vi "Add Snake Class.vi"(8 "error in (no error)":errorcluster, 10 "Snake":refnum<class "Snake.lvclass">, 11 "Board_Game in":refnum<class "Board_Game.lvclass">) -> (0 "error out":errorcluster, 3 "Board_Game out":refnum<class "Board_Game.lvclass">)   [LabVIEW 2021, in "Board_Game.lvclass"]
uses:
  Board_Game.lvclass
  SnakeGame/Snake.lvclass
  Direction.ctl
  Board_Game.lvclass/Board_Game.ctl
  SnakeGame/Position.ctl
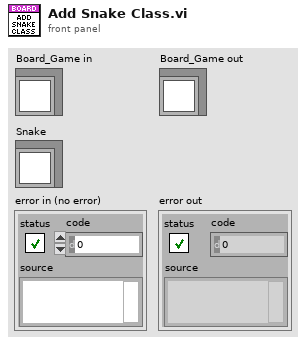
[diagram p1: front panel]
types:
  T1 = typedef "Direction.ctl" = enum16{"Up", "Down", "Left", "Right"}
  T2 = typedef "Position.ctl" = cluster{"X":u32, "Y":u32}
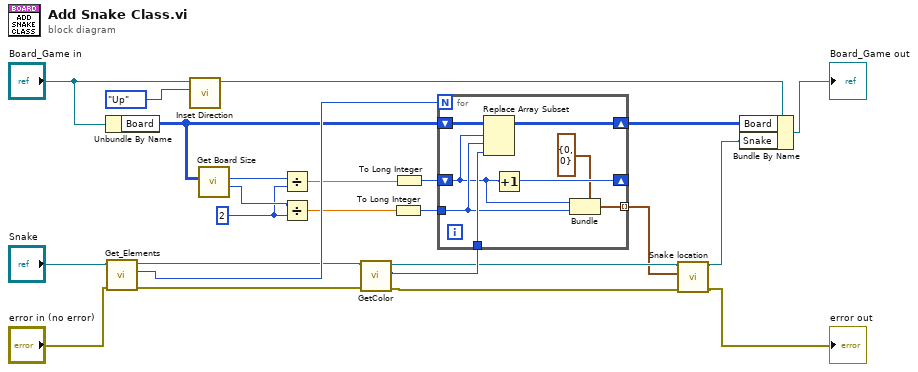
[diagram p0: block diagram]
diagram:
  w8 = 2 ("y")
  n1 = Unbundle By Name("Board_Game in") -> ("Board"=w13:u32[][])
  n2 = call-dynamic "Get_Elements.vi"("error in (no error)"="error in (no error)", "Snake in"="Snake") -> ("error out"=w5:errorcluster, "Start Elements"=w17:u32, "Snake out"=w16:refnum<class "Snake.lvclass">)  [unwired: 7 in]
  n3 = call-dynamic "Inset Direction.vi"("Keyboard"=Direction."Up", "Board_Game in"="Board_Game in") -> ("Board_Game out"=w22:refnum<class "Board_Game.lvclass">)  [unwired: 8 in, 1 out]
  n4 = call "Get Board Size.vi"("Board"=w13) -> ("Y"=w9:i32, "X"=w12:i32)  [unwired: 9 in]
  n5 = Divide(x=w12, y=w8) -> (x/y=w11:dbl)
  n6 = Divide(x=w9, y=w8) -> (x/y=w10:dbl)
  n7 = call-dynamic "GetColor.vi"("error in (no error)"=w5, "SnakeGame in"=w16) -> ("error out"=w3:errorcluster, "Color"=w14:u32, "SnakeGame out"=w7:refnum<class "Snake.lvclass">)  [unwired: 7 in]
  n8 = To Long Integer(number=w10) -> (32bit integer=w18:i32)
  n9 = To Long Integer(number=w11) -> (32bit integer=w19:i32)
  n10 = for {
    N: w17 -> [_]
    shift-right: [w32] -> w15
    shift-left: w13 -> [w31]
    tunnel: w14 -> [w30]
    shift-right: [w29] -> _
    shift-left: w19 -> [w26]
    tunnel: w18 -> [w27]
    tunnel: [w25] -> w1 mode=indexing
    n11 = Replace Array Subset(array=w31, new element=w30, index (row)=w26, index (col)=w27) -> (w32:u32[][])
    n12 = Increment(x=w26) -> (x+1=w29:i32)
    n13 = Bundle(cluster=T2 {"X"=0, "Y"=0} ("Position"), "X"=w26, "Y"=w27) -> (w25:T2)
  }
  n14 = call-dynamic "Snake location.vi"("error in (no error)"=w3, "Snake location"=w1, "Snake in"=w7) -> ("error out"=→"error out":errorcluster, "Snake out"=w6:refnum<class "Snake.lvclass">)  [unwired: 7 in]
  n15 = Bundle By Name(cluster=w22, "Board"=w15, "Snake"=w6) -> (→"Board_Game out":refnum<class "Board_Game.lvclass">)
